vi "Control Value Variant From Registry.vi"(4 "Registry Variant Accessor (optional)":refnum<class "CConfig Variant Accessor.lvclass">, 6 "Controls":refnum<vi>[](array[refnum]), 7 "Registry Control Reference Accessor (optional)":refnum<class "Registry Ctrl Ref Accessor.lvclass">, 8 "error in (no error)":errorcluster, 9 "Use LV Default? [F]":bool, 11 "Registry Object in":refnum<class "Carya Config.lvclass">) -> (0 "error out":errorcluster, 1 "Used controls":refnum<vi>[](array[refnum]), 2 "Used variants":variant[](array[variant]), 3 "Registry Object out":refnum<class "Carya Config.lvclass">)   [LabVIEW 2013, in "Carya Config.lvclass"]
doc: "Copyright 2018, Carya Automatisering, Wiebe Walstra."
uses:
  Carya Config.lvclass
  CConfig Ctrl Ref Accessor/Registry Ctrl Ref Accessor.lvclass
  CConfig Variant Accessor/CConfig Variant Accessor.lvclass
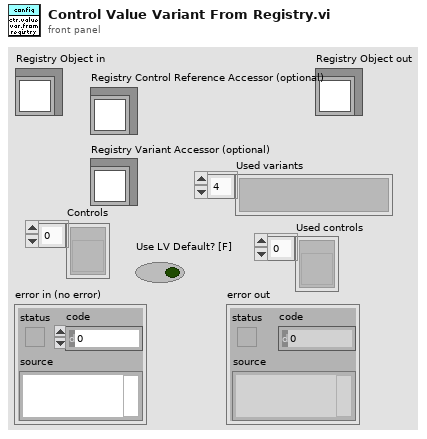
[diagram p1: front panel]
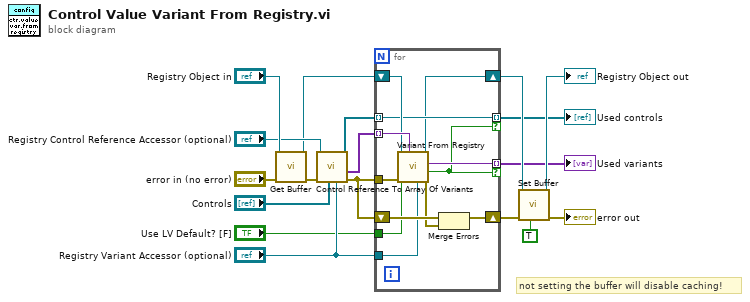
[diagram p0: block diagram]
diagram:
  # "not setting the buffer will disable caching!"
  n1 = call-dynamic "Get Buffer.vi"("error in (no error)"="error in (no error)", "Carya Config in"="Registry Object in") -> ("error out"=w5:errorcluster, "Config"=w7:refnum<class "Carya Config.lvclass">)  [unwired: 8 in]
  n2 = call-dynamic "Control Reference To Array Of Variants.vi"("Registry Variant Accessor"="Registry Variant Accessor (optional)", "Controls"="Controls", "error in (no error)"=w5, "Registry Control Reference Accessor in"="Registry Control Reference Accessor (optional)") -> ("error out"=w3:errorcluster, "Variants"=w13:variant[], "Controls"=w10:refnum<vi>[])  [unwired: 4 in, 1 out]
  n3 = for {
    tunnel: w3 -> [w30]
    tunnel: w13 -> [w29] mode=indexing
    tunnel: "Registry Variant Accessor (optional)" -> [w21]
    shift-right: [w27] -> w2
    shift-left: w3 -> [w28]
    shift-right: [w22] -> w8
    shift-left: w7 -> [w24]
    tunnel: w10 -> [w23] mode=indexing
    tunnel: "Use LV Default? [F]" -> [w25]
    tunnel: [w23] -> w6 mode=indexing if=w19
    tunnel: [w20] -> w1 mode=indexing if=w19
    n4 = call "Variant From Registry.vi"("Registry Variant Accessor in"=w21, "Variant"=w29, "error in (no error)"=w30, "Use LV Default? [F]"=w25, "Carya Config in"=w24) -> ("error out"=w26:errorcluster, "Set?"=w19:bool, "Variant"=w20:variant, "Carya Config out"=w22:refnum<class "Carya Config.lvclass">)  [unwired: 3 in]
    n5 = Merge Errors(w28, w26) -> (w27:errorcluster)
  }
  "Used controls" <- w6
  "Used variants" <- w1
  n6 = call-dynamic "Set Buffer.vi"("Set? [T]"=TRUE, "error in (no error)"=w2, "Carya Config"=w8) -> ("error out"=→"error out":errorcluster, "Carya Config out"=→"Registry Object out":refnum<class "Carya Config.lvclass">)  [unwired: 7 in]
